vi "State calculator.vi"(5 "Current loop \nnumber":i16, 7 "Trigger":bool, 9 "wait time":sgl, 11 "hw cal time":sgl) -> (8 "State":i8)   [LabVIEW 2019]
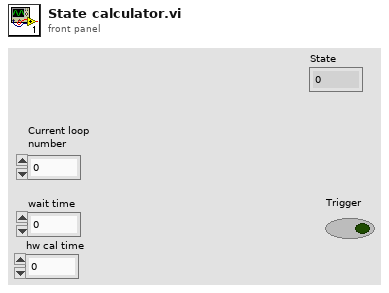
[diagram p1: front panel]
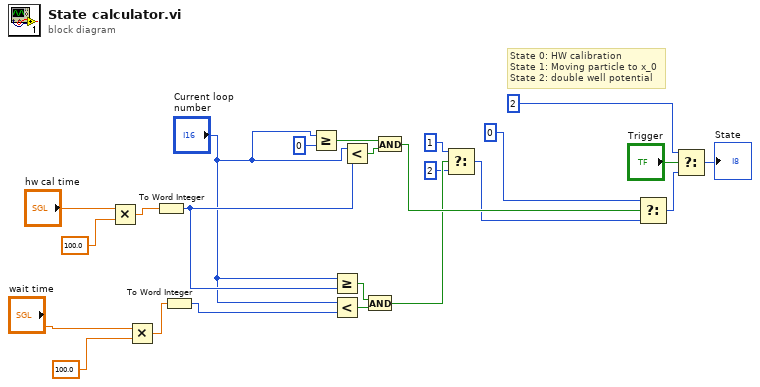
[diagram p0: block diagram]
diagram:
  # "State 0: HW calibration\nState 1: Moving particle to x_0\nState 2: double well potential"
  n1 = Multiply(x="hw cal time", y=sgl 100.0) -> (x*y=w19:sgl)
  n2 = Multiply(x="wait time", y=sgl 100.0) -> (x*y=w13:sgl)
  n3 = To Word Integer(number=w19) -> (16bit integer=w14:i16)
  n4 = To Word Integer(number=w13) -> (16bit integer=w12:i16)
  n5 = Greater Or Equal?(x="Current loop \nnumber", y=i16 0) -> (x >= y?=w18:bool)
  n6 = Greater Or Equal?(x="Current loop \nnumber", y=w14) -> (x >= y?=w16:bool)
  n7 = Less?(x="Current loop \nnumber", y=w12) -> (x < y?=w15:bool)
  n8 = Less?(x="Current loop \nnumber", y=w14) -> (x < y?=w17:bool)
  n9 = And(x=w16, y=w15) -> (x .and. y?=w8:bool)
  n10 = And(x=w18, y=w17) -> (x .and. y?=w10:bool)
  n11 = Select(t=i8 1, s=w8, f=i8 2) -> (s? t:f=w7:i8)
  n12 = Select(t=i8 0, s=w10, f=w7) -> (s? t:f=w2:i8)
  n13 = Select(t=i8 2, s="Trigger", f=w2) -> (s? t:f=→"State":i8)
